vi "DataLog-Flush.vi"(0 "state":T1, 11 "error in (no error)":errorcluster) -> (15 "error out":errorcluster)   [LabVIEW 2020]
uses:
  DataLog-State.ctl
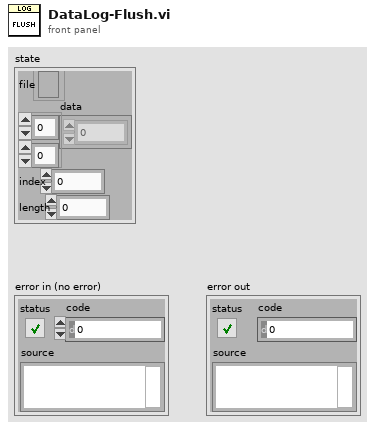
[diagram p1: front panel]
types:
  T1 = typedef "DataLog-State.ctl" = cluster{"file":refnum<file>, "data":dbl[][], "index":i32, "length":i32}
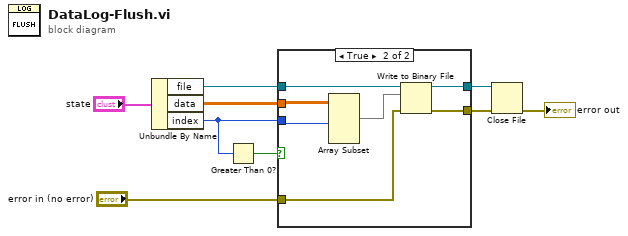
[diagram p0: block diagram]
diagram:
  n1 = Unbundle By Name("state") -> ("file"=w5:refnum<file>, "data"=w6:dbl[][], "index"=w7:i32)
  n2 = Greater Than 0?(x=w7) -> (x > 0?=w8:bool)
  n3 = case shown="True" w8 {
    tunnel: w7 -> [_ w17]
    tunnel: w6 -> [_ w18]
    tunnel: w5 -> [w11 w16]
    tunnel: [w11 w14] -> w2
    tunnel: "error in (no error)" -> [w10 w13]
    tunnel: [w10 w12] -> w3
    frame False {
    }
    frame True {
      n4 = Array Subset(array=w18, length (row)=w17) -> (w15:dbl[][])  [unwired: 3 in]
      n5 = Write to Binary File(file (use dialog)=w16, data=w15, error in=w13) -> (refnum out=w14:refnum<file>, error out=w12:errorcluster)  [unwired: 3 in, 1 out]
    }
  }
  n6 = Close File(refnum=w2, error in=w3) -> (error out=→"error out":errorcluster)  [unwired: 1 out]
